vi "ExpandBuffer.vi"(8 "error in (no error)":errorcluster, 11 "BufferedArray in":refnum<class "BufferedArray.lvclass">) -> (0 "error out":errorcluster, 3 "BufferedArray out":refnum<class "BufferedArray.lvclass">)   [LabVIEW 2013, in "LapDog.Collections.v1.Lists.Implementations.lvlib" / "BufferedArray.lvclass"]
doc: "Increase the size of the buffer. If buffer size < MaxInc, double the size. Otherwise increase buffer by MaxInc."
uses:
  BufferedArray.lvclass
  BufferedArray.lvclass/BufferedArray.ctl
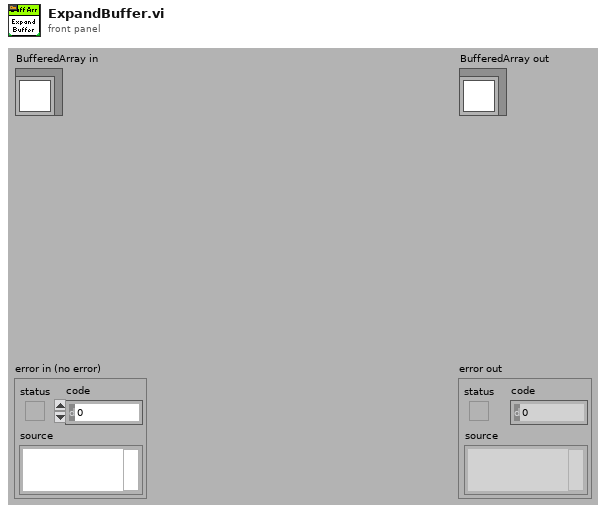
[diagram p1: front panel]
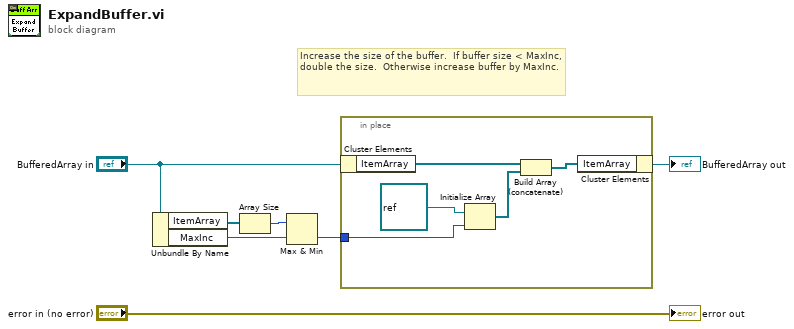
[diagram p0: block diagram]
diagram:
  # "Increase the size of the buffer.  If buffer size < MaxInc, double the size.  Otherwise increase buffer by MaxInc."
  n1 = Unbundle By Name("BufferedArray in") -> ("ItemArray"=w5:refnum<class>[], "MaxInc"=w3:i32)
  n2 = Array Size(array=w5) -> (size(s)=w4:i32)
  n3 = Max & Min(x=w4, y=w3) -> (min(x,y)=w1:i32)  [unwired: 1 out]
  n4 = in-place {
    in-place-border: w1 -> [w8]
    n5 = in-place-cluster #1("BufferedArray in") -> ("ItemArray"=w10:refnum<class>[])
    n6 = Initialize Array(refnum<class> refnum ("LabVIEW Object"), w8) -> (w11:refnum<class>[])
    n7 = Build Array (concatenate)(w10, w11) -> (w9:refnum<class>[])
    n8 = in-place-cluster #1("ItemArray"=w9) -> (→"BufferedArray out":refnum<class "BufferedArray.lvclass">)
  }
  "error out" <- "error in (no error)"
